vi "TIO Stream Read Non-blocking.vi"(8 "error in (no error)":errorcluster, 11 "TC Connection":T1={"Type"=enum."Serial", "URL"="serial:///dev/cu.usbserial-00000", "TO"=500, "Addr"=0, "Port"=0, "TCP"=refnum, "UDP"=refnum, "Route"=""}) -> (0 "error out":errorcluster, 1 "Payload":string, 2 "Type":u16(ring)=2 items=["Invalid", "Log", "RPC Request", "RPC Reply", "RPC Error", "Stream Description", "User"], 3 "TC Connection":T1={"Type"=enum."Serial", "URL"="serial:///dev/cu.usbserial-00000", "TO"=500, "Addr"=0, "Port"=0, "TCP"=refnum, "UDP"=refnum, "Route"=""}, 4 "Route":string, 5 "Routing Matches":bool)   [LabVIEW 2020]
uses:
  <instrlib>/tio-labview/TIO Library/TIO Serial Checksum CRC32.vi
panel:
  out "Routing Size":u8
  out "Payload Length":u16
  # "TODO Handle routing"
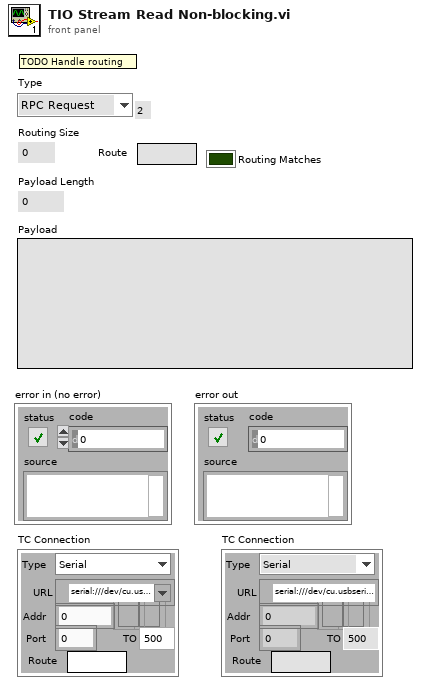
[diagram p1: front panel]
types:
  T1 = cluster{"Type":enum16{"Serial", "TCP", "UDP", "mUDP"}, "URL":refnum<visa-resource-name>, "TO":u32, "Addr":u32, "Port":i32, "TCP":refnum<k5>, "UDP":refnum<k16>, "Route":string}
  T2 = enum16{"Standard", "Buffered", "CRLF", "Immediate"}
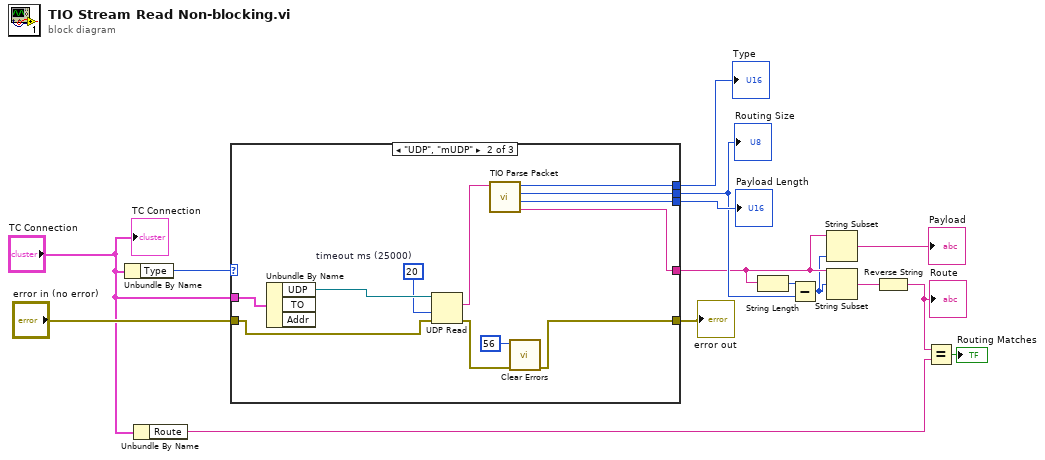
[diagram p0: block diagram]
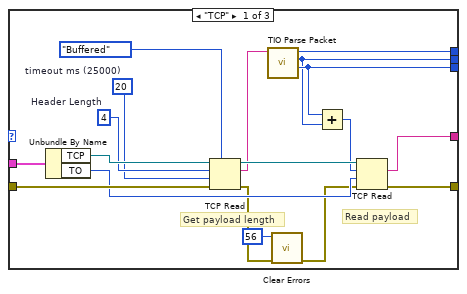
[diagram p2: hidden frame]
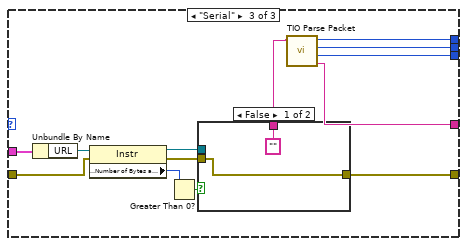
[diagram p3: hidden frame]
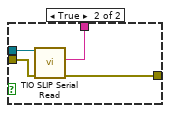
[diagram p4: hidden frame]
diagram:
  n1 = Unbundle By Name("TC Connection") -> ("Type"=w13:enum16{"Serial", "TCP", "UDP", "mUDP"})
  n2 = Unbundle By Name("TC Connection") -> ("Route"=w4:string)
  n3 = case shown="\"UDP\", \"mUDP\"" w13 {
    tunnel: "error in (no error)" -> [w30 w34 w49]
    tunnel: [w29 w35 w58] -> w15
    tunnel: "TC Connection" -> [w33 w45 w57]
    tunnel: [w28 w38 w53] -> w8
    tunnel: [w18 w43 w54] -> w12
    tunnel: [w17 w42 w55] -> w9
    tunnel: [w24 w44 w56] -> w11
    frame "TCP" {
      w23 = 20  # timeout ms (25000)
      w26 = u32 4  # Header Length
      # "Read payload"
      # "Get payload length"
      n4 = Unbundle By Name(w33) -> ("TCP"=w32:refnum<k5>, "TO"=w27:u32)
      n5 = TCP Read(connection ID=w32, bytes to read=w26, error in (no error)=w30, 7:T2."Buffered" ("mode (standard)"), 9:w23) -> (connection ID out=w31:refnum<k5>, data out=w25:string, error out=w21:errorcluster)
      n6 = call <instrlib>:"TIO Parse Packet.vi"("Packet"=w25) -> ("Payload Length"=w18:u16, "Routing Size"=w17:u8, "Type"=w24:u16)  [unwired: 7 in, 1 out]
      n7 = call <vilib>:"Clear Errors.vi"("error in (no error)"=w21, "specific error code to clear (0: all)"=56) -> ("error out"=w20:errorcluster)  [unwired: 4 in, 1 out]
      n8 = Add(x=w18, y=w17) -> (x+y=w16:u16)
      n9 = TCP Read(connection ID=w31, bytes to read=w16, error in (no error)=w20, 9:w27) -> (data out=w28:string, error out=w29:errorcluster)  [unwired: 1 in, 1 out]
    }
    frame "UDP", "mUDP" {
      w40 = 20  # timeout ms (25000)
      n10 = Unbundle By Name(w45) -> ("UDP"=w41:refnum<k16>)  [unwired: 2 out]
      n11 = UDP Read(connection ID=w41, timeout ms (25000)=w40, 8:w34) -> (data out=w39:string, error out=w36:errorcluster)  [unwired: 1 in, 3 out]
      n12 = call <instrlib>:"TIO Parse Packet.vi"("Packet"=w39) -> ("Payload"=w38:string, "Payload Length"=w43:u16, "Routing Size"=w42:u8, "Type"=w44:u16)  [unwired: 7 in]
      n13 = call <vilib>:"Clear Errors.vi"("error in (no error)"=w36, "specific error code to clear (0: all)"=56) -> ("error out"=w35:errorcluster)  [unwired: 4 in, 1 out]
    }
    frame "Serial" {
      n14 = Unbundle By Name(w57) -> ("URL"=w51:refnum<visa-resource-name>)
      n15 = property class="Instr"(reference=w51, error in=w49) -> (reference out=w50:refnum<visa-resource-name>, error out=w48:errorcluster, "Serial Settings:Number of Bytes at Serial Port"=w47:u32)
      n16 = Greater Than 0?(x=w47) -> (x > 0?=w46:bool)
      n17 = case shown="False" w46 {
        tunnel: [w60 w64] -> w58
        tunnel: ["" ("Payload") w63] -> w52
        tunnel: w50 -> [_ w62]
        tunnel: w48 -> [w60 w61]
        frame False {
        }
        frame True {
          n18 = call <instrlib>:"TIO SLIP Serial Read.vi"("error in (no error)"=w61, "VISA resource name"=w62) -> ("error out"=w64:errorcluster, "Payload"=w63:string)  [unwired: 7 in, 1 out]
        }
      }
      n19 = call <instrlib>:"TIO Parse Packet.vi"("Packet"=w52) -> ("Payload"=w53:string, "Payload Length"=w54:u16, "Routing Size"=w55:u8, "Type"=w56:u16)  [unwired: 7 in]
    }
  }
  "error out" <- w15
  "Type" <- w11
  "Routing Size" <- w9
  "Payload Length" <- w12
  n20 = String Length(string=w8) -> (length=w10:i32)
  n21 = Subtract(x=w10, y=w9) -> (x-y=w7:i32)
  n22 = String Subset(string=w8, length (rest)=w7) -> (substring=→"Payload":string)  [unwired: 1 in]
  n23 = String Subset(string=w8, offset (0)=w7) -> (substring=w2:string)  [unwired: 1 in]
  n24 = Reverse String(1:w2) -> (0:w1:string)
  "Route" <- w1
  n25 = Equal?(x=w1, y=w4) -> (x = y?=→"Routing Matches":bool)
  "TC Connection" <- "TC Connection"
